vi "Tell Reply.vi"(4 "Priority":bool, 6 "Teller":refnum<class "Teller.lvclass">, 7 "Actor in":refnum<class "Actor.lvclass">, 9 "Parent Stopped":bool, 10 "Safe Stop":bool=TRUE) -> (0 "Error out":errorcluster)   [LabVIEW 2025, in "jettl.lvlib" / "Stop Msg.lvlib"]
uses:
  Stop Msg.lvlib
  Teller/Teller/Teller.lvclass
  Actor/Actor.lvclass
  Stop Msg/Stop Msg.lvclass
  C:/git/jettl/src/jettl/jettl/Msg/Msg.lvclass
  jettl.lvlib
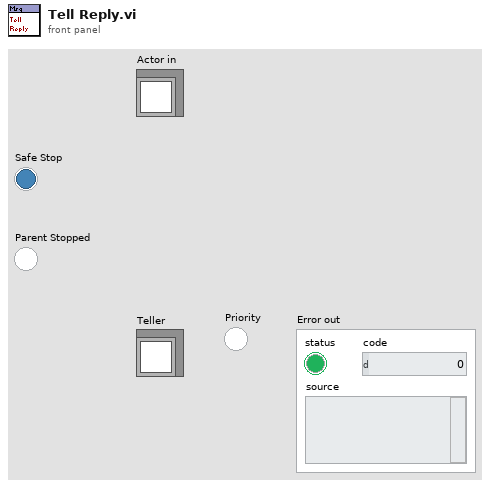
[diagram p1: front panel]
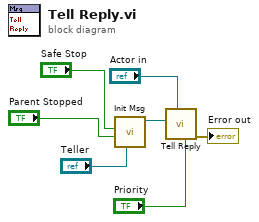
[diagram p0: block diagram]
diagram:
  n1 = call "Init Msg.vi"("Teller"="Teller", "Parent Stopped"="Parent Stopped", "Safe Stop"="Safe Stop") -> ("Stop Msg out"=w3:refnum<class "Stop Msg.lvclass">)  [unwired: 8 in]
  n2 = call "Tell Reply.vi"("Priority"="Priority", "Actor in"="Actor in", "Msg"=w3) -> ("Error out"=→"Error out":errorcluster)  [unwired: 8 in]
